vi "TSM Relay Expand Action Array to All Sessions.vi"(0 "TSM Relay in":T2={"TSM context"=refnum, "Pin Query Context"=refnum, "TSM Site Numbers"=[], "SSC Relay"=[], "Unfiltered Pins"=[], "Filtered Pins"=[], "Filtered Pins Info"={"Unfiltered Pins Count"=3, "Locations"=[], "Lengths"=[]}}, 7 "Relay Actions in":T5[](array[typedef]) items=["Open Relay"=20, "Close Relay"=21]) -> (4 "SSC Relay":T1[](array[typedef]), 8 "Expanded Relay Actions":T5[](array[typedef]) items=["Open Relay"=20, "Close Relay"=21], 15 "Filtered Pins":string[](array[string]))   [LabVIEW 2019]
doc: "This VI expands the Relay Actions to each SSC Relay session based on Pin Grouping from the Filtered Pins."
uses:
  <instrlib>/niSwitch/niSwitch.llb/niSwitch Relay Action.ctl
  TSM SSC Relay.ctl
  <vilib>/NI_TestStand_SemiconductorModule/NI_TestStand_Semiconductor_Module.lvlibp/PinMap/PinQueryContext/MultiplePinMultipleSessionQueryContext/MultiplePinMultipleSessionQueryContext.lvclass
  <vilib>/NI_TestStand_SemiconductorModule/NI_TestStand_Semiconductor_Module.lvlibp/PinMap/General/SemiconductorModuleContext.ctl
  SSC/SSC Relay.ctl
  TSM Filtered Pins Info.ctl
  <vilib>/NI_TestStand_SemiconductorModule/NI_TestStand_Semiconductor_Module.lvlibp
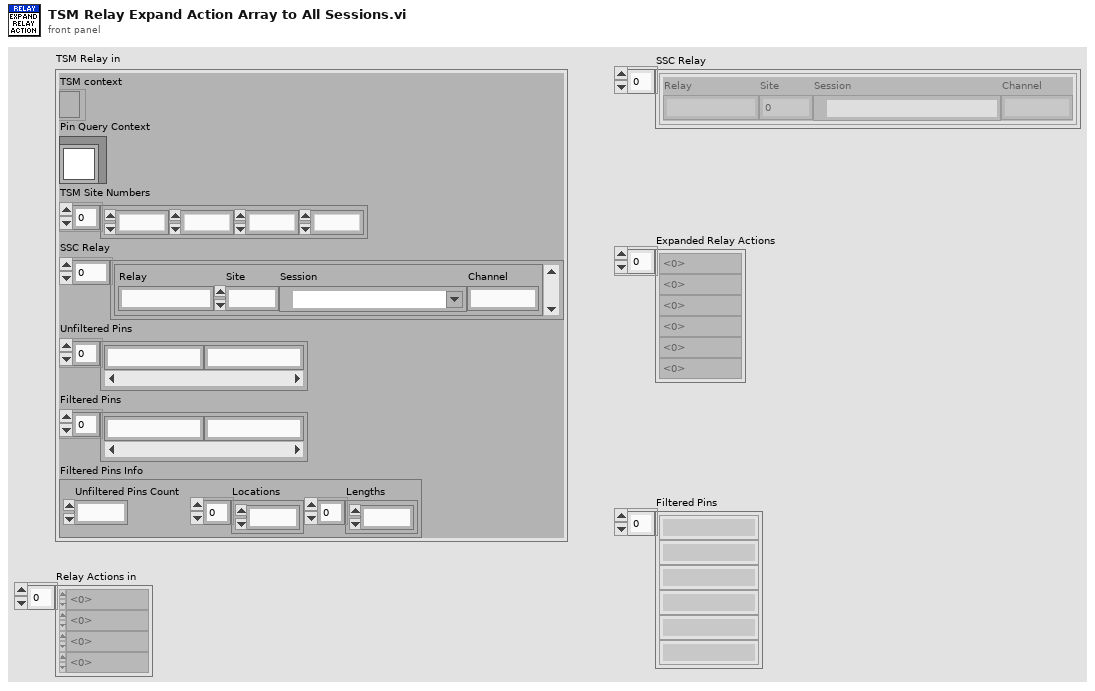
[diagram p1: front panel]
types:
  T1 = typedef "SSC Relay.ctl" = cluster{"Relay":string, "Site":i32, "Session":refnum<k15>, "Channel":string}
  T2 = typedef "TSM SSC Relay.ctl" = cluster{"TSM context":T3, "Pin Query Context":refnum<class "MultiplePinMultipleSessionQueryContext.lvclass">, "TSM Site Numbers":i32[], "SSC Relay":T1[], "Unfiltered Pins":string[], "Filtered Pins":string[], "Filtered Pins Info":T4}
  T3 = typedef "NI_TestStand_Semiconductor_Module.lvlibp/SemiconductorModuleContext.ctl" = refnum<k7>
  T4 = typedef "TSM Filtered Pins Info.ctl" = cluster{"Unfiltered Pins Count":i32, "Locations":i32[], "Lengths":i32[]}
  T5 = typedef "niSwitch Relay Action.ctl" = i32
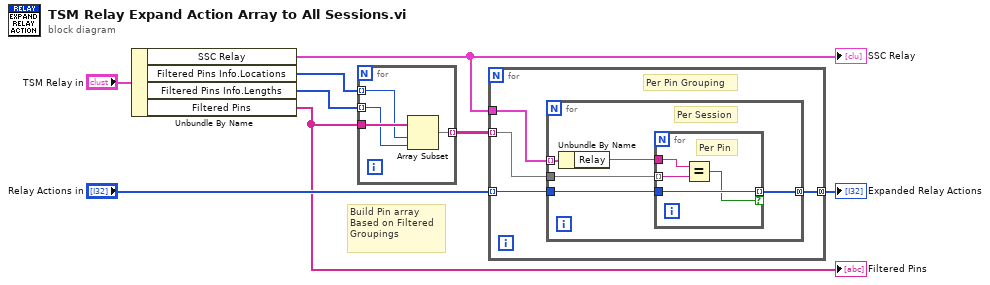
[diagram p0: block diagram]
diagram:
  # "Build Pin array Based on Filtered Groupings"
  n1 = Unbundle By Name("TSM Relay in") -> ("SSC Relay"=w1:T1[], "Filtered Pins Info.Locations"=w6:i32[], "Filtered Pins Info.Lengths"=w7:i32[], "Filtered Pins"=w2:string[])
  "Filtered Pins" <- w2
  "SSC Relay" <- w1
  n2 = for {
    tunnel: w6 -> [w11] mode=indexing
    tunnel: w7 -> [w10] mode=indexing
    tunnel: w2 -> [w12]
    tunnel: [w9] -> w8 mode=indexing
    n3 = Array Subset(array=w12, index=w11, length=w10) -> (w9:string[])
  }
  n4 = for {
    tunnel: w1 -> [w16]
    tunnel: [w15] -> w5 mode=concatenating
    tunnel: "Relay Actions in" -> [w14] mode=indexing
    tunnel: w8 -> [w13] mode=indexing
    # "Per Pin Grouping"
    n5 = for {
      tunnel: w16 -> [w21] mode=indexing
      tunnel: w14 -> [w19]
      tunnel: [w18] -> w15 mode=concatenating
      tunnel: w13 -> [w17]
      # "Per Session"
      n6 = Unbundle By Name(w21) -> ("Relay"=w20:string)
      n7 = for {
        tunnel: w20 -> [w25]
        tunnel: w19 -> [w24]
        tunnel: [w24] -> w18 mode=indexing if=w23
        tunnel: w17 -> [w22] mode=indexing
        # "Per Pin"
        n8 = Equal?(x=w25, y=w22) -> (x = y?=w23:bool)
      }
    }
  }
  "Expanded Relay Actions" <- w5
